vi "test_example.vi"   [LabVIEW 2020]
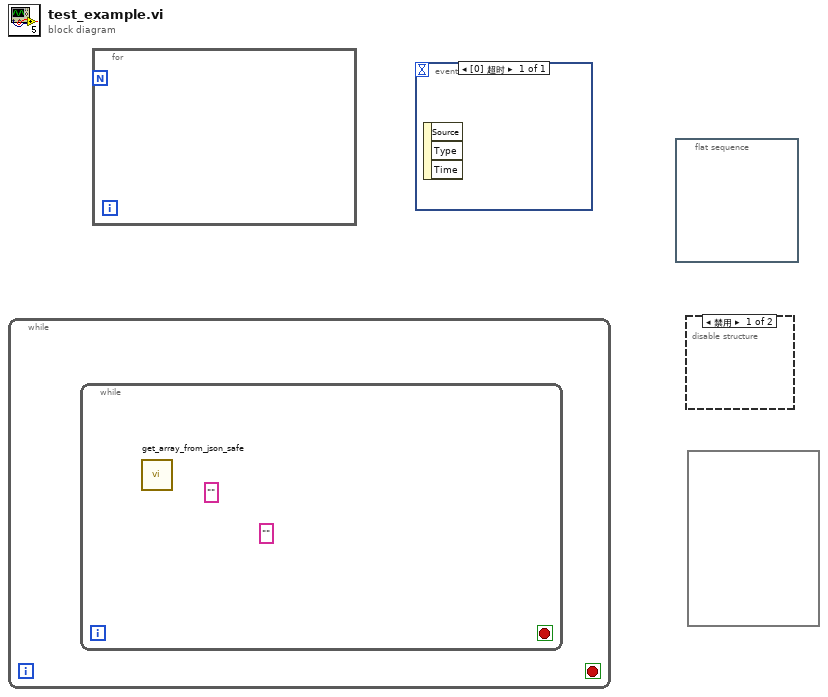
[diagram p0: block diagram]
diagram:
  n1 = while {
    stop <- _ stop-if-true
    n2 = while {
      stop <- _ stop-if-true
      (unwired) ""
      (unwired) ""
      n3 = call "get_array_from_json_safe.vi"() -> ()  [unwired: 11 in, 1 out]
    }
  }
  n4 = for {
  }
  n5 = event shown="[0] 超时" {
    selector: _ -> [_]
    dyn-events: _ -> [_]
    timeout: _ -> [_]
    event Timeout {
      n6 = event-data() -> ()  [unwired: 1 in, 3 out]
    }
  }
  n7 = flat-sequence {
    frame #0 {
    }
  }
  n8 = disable-structure shown="禁用" {
    frame Disabled {
    }
    frame Enabled {
    }
  }
  n9 = formula code=""() -> ()
